vi "Read Power Over Coax Voltage and Current.vi"(0 "fpga interface in":refnum<k20>, 5 "serial channels":string[](array[string]), 11 "error in (no error)":errorcluster) -> (4 "fpga interface out":refnum<k20>, 6 "current (A)":dbl[](array[numeric]), 8 "voltage (V)":dbl[](array[numeric]), 10 "in range":bool[](array[boolean]), 15 "error out":errorcluster)   [LabVIEW 2023, in "GettingStarted_Common_148X_Host.lvlib"]
uses:
  GettingStarted_Common_148X_Host.lvlib
  <instrlib>/FlexRIO/API/Host/v1/NI FlexRIO/API/Get Property Reference - Fpga Small.vi
  <instrlib>/FlexRIO/API/Host/v1/NI FlexRIO API v1.lvlib
  <resource>/objmgr/niflexrioapiChannel.rc
  <instrlib>/FlexRIO/Automotive Vision Utility/v1/Host/Automotive Vision Utility.lvlib
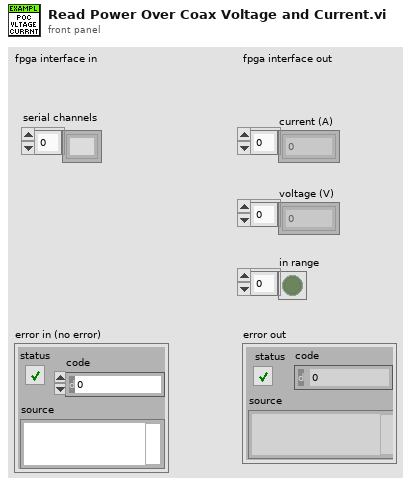
[diagram p1: front panel]
types:
  T1 = typedef "Automotive Vision Utility.lvlib/Serial Channel Type.ctl" = enum16{"Serial Input Channel", "Serial Output Channel", "Unknown Channel Type"}
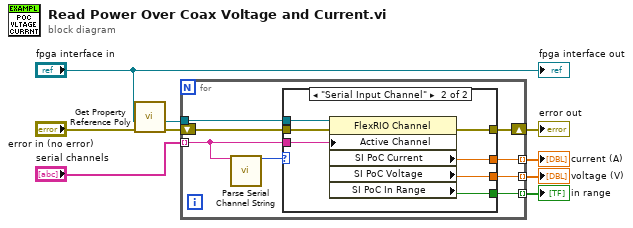
[diagram p0: block diagram]
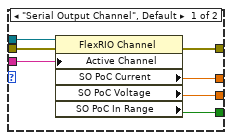
[diagram p2: hidden frame]
diagram:
  n1 = call-poly <instrlib>:"Get Property Reference Poly.vi"("error in (no error)"="error in (no error)", "fpga interface in"="fpga interface in") -> ("error out"=w3:errorcluster, "property reference"=w2:refnum<k20>)  [unwired: 4 in, 1 out]
  n2 = for {
    tunnel: "serial channels" -> [w14] mode=indexing
    shift-right: [w17] -> w9
    shift-left: w3 -> [w15]
    tunnel: w2 -> [w16]
    tunnel: [w12] -> w7 mode=indexing
    tunnel: [w11] -> w8 mode=indexing
    tunnel: [w10] -> w1 mode=indexing
    n3 = call <instrlib>:"Parse Serial Channel String.vi"("serial channel string"=w14) -> ("serial channel type"=w13:T1)  [unwired: 13 in, 1 out]
    n4 = case shown="\"Serial Input Channel\"" w13 {
      tunnel: [w22 w31] -> w17
      tunnel: w14 -> [w21 w30]
      tunnel: w16 -> [w24 w29]
      tunnel: w15 -> [w23 w28]
      tunnel: [w19 w27] -> w12
      tunnel: [w20 w26] -> w11
      tunnel: [w18 w25] -> w10
      frame "Serial Output Channel", Default {
        n5 = property class="FlexRIO Channel"(reference=w24, error in=w23, "Active Channel"=w21) -> (error out=w22:errorcluster, "SO PoC Current"=w19:dbl, "SO PoC Voltage"=w20:dbl, "SO PoC In Range"=w18:bool)  [unwired: 1 out]
      }
      frame "Serial Input Channel" {
        n6 = property class="FlexRIO Channel"(reference=w29, error in=w28, "Active Channel"=w30) -> (error out=w31:errorcluster, "SI PoC Current"=w27:dbl, "SI PoC Voltage"=w26:dbl, "SI PoC In Range"=w25:bool)  [unwired: 1 out]
      }
    }
  }
  "error out" <- w9
  "current (A)" <- w7
  "voltage (V)" <- w8
  "in range" <- w1
  "fpga interface out" <- "fpga interface in"
